vi "norm dist rand num.vi"(1 "Numeric 2":dbl) -> (0 "Numeric":dbl)   [LabVIEW 2010]
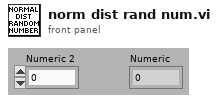
[diagram p1: front panel]
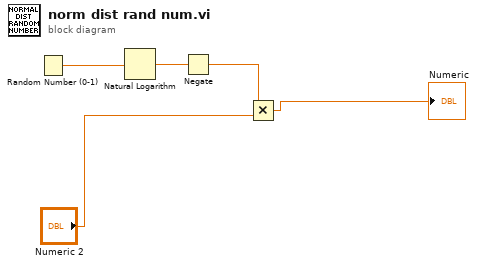
[diagram p0: block diagram]
diagram:
  n1 = Random Number (0-1)() -> (number: 0 to 1=w1:dbl)
  n2 = Natural Logarithm(1:w1) -> (0:w2:dbl)
  n3 = Negate(x=w2) -> (-x=w3:dbl)
  n4 = Multiply(x=w3, y="Numeric 2") -> (x*y=→"Numeric":dbl)
